vi "Resolve Direction Position.vi"(7 "Board Size":i32, 10 "Direction":T1, 11 "From":T2) -> (2 "Col":i32, 3 "Row":i32, 5 "To":T2)   [LabVIEW 2020, in "SquareBattle.lvlib"]
doc: "Returns the position that is the specified direction from the specified starting position. The board size must also be provided to handle wrapping around board edges."
uses:
  SquareBattle.lvlib
  Position.ctl
  Direction.ctl
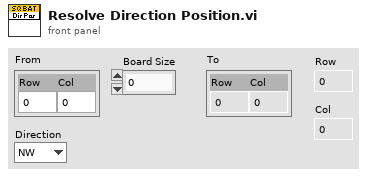
[diagram p1: front panel]
types:
  T1 = typedef "SquareBattle.lvlib/Direction.ctl" = enum16{"NW", "N", "NE", "E", "SE", "S", "SW", "W"}
  T2 = typedef "SquareBattle.lvlib/Position.ctl" = cluster{"Row":i32, "Col":i32}
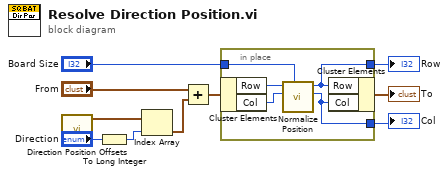
[diagram p0: block diagram]
diagram:
  n1 = call "Direction Position Offsets.vi"() -> ("Direction Position Offsets"=w9:T2[])  [unwired: 11 in]
  n2 = To Long Integer(number="Direction") -> (32bit integer=w8:i32)
  n3 = Index Array(array=w9, index=w8) -> (element=w7:T2)
  n4 = Add(x="From", y=w7) -> (x+y=w5:T2)
  n5 = in-place {
    in-place-border: "Board Size" -> [w13]
    in-place-border: [w11] -> w2
    in-place-border: [w12] -> w1
    n6 = in-place-cluster #1(w5) -> ("Row"=w15:i32, "Col"=w14:i32)
    n7 = call "Normalize Position.vi"("Size"=w13, "Col In"=w14, "Row In"=w15) -> ("Col"=w11:i32, "Row"=w12:i32)  [unwired: 7 in]
    n8 = in-place-cluster #1("Row"=w12, "Col"=w11) -> (→"To":T2)
  }
  "Col" <- w2
  "Row" <- w1
